vi "Set Receiver.vi"(8 "error in (no error)":errorcluster caption="错误输入（无错误）", 10 "Receiver":string, 11 "Message输入":refnum<class "Message.lvclass">) -> (0 "error out":errorcluster caption="错误输出", 3 "Message输出":refnum<class "Message.lvclass">)   [LabVIEW 2011, in "Message.lvclass"]
uses:
  Message.lvclass
  Message.lvclass/Message.ctl
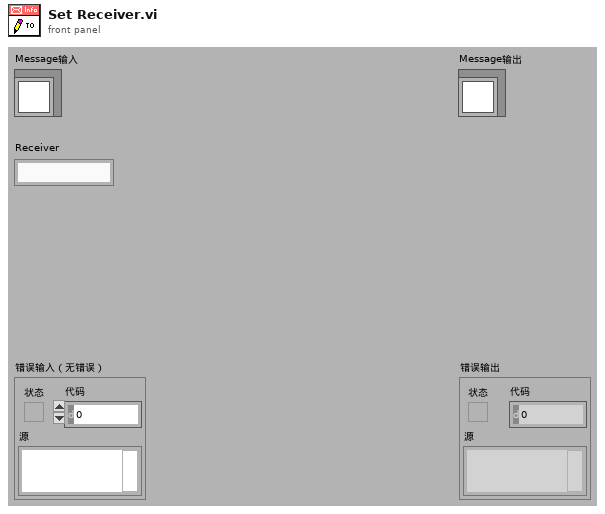
[diagram p1: front panel]
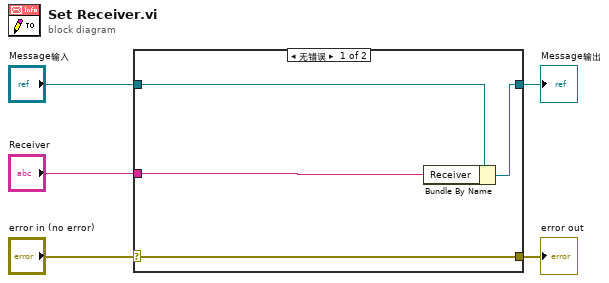
[diagram p0: block diagram]
diagram:
  n1 = case shown="无错误" "error in (no error)" {
    selector: "error in (no error)" -> [w9 w10]
    tunnel: [w9 w10] -> w4
    tunnel: [w7 w11] -> w2
    tunnel: "Message输入" -> [w8 w11]
    tunnel: "Receiver" -> [w6 _]
    frame No Error {
      n2 = Bundle By Name(cluster=w8, "Receiver"=w6) -> (w7:refnum<class "Message.lvclass">)
    }
    frame Error {
    }
  }
  "error out" <- w4
  "Message输出" <- w2
